vi "PH_IEEE1394Camera.get Cam Video Modes.vi"(0 "i ref in":refnum<vi>, 2 "IMAQ1394 Session In":T1, 4 "Cam Error in":errorcluster, 5 "error in (no error)":errorcluster) -> (14 "i ref out":refnum<vi>, 16 "IMAQ1394 Session Out":T1, 18 "Cam Error out":errorcluster, 19 "error out":errorcluster)   [LabVIEW 2014, in "PH_IEEE1394Camera.lvlib"]
doc: "This VI gets the video modes and sets them to the GUI and own attributes."
uses:
  PH_IEEE1394Camera.lvlib
  <vilib>/userdefined/High Color/IMAQdx.ctl
  <vilib>/vision/driver/NI_Vision_Acquisition_Software.lvlib
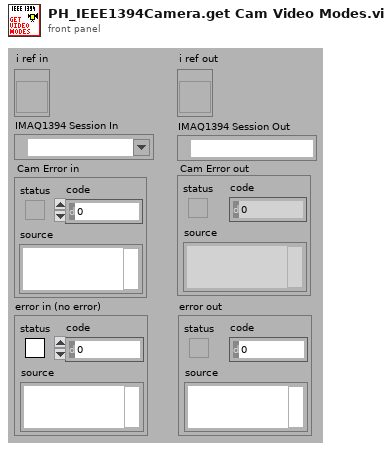
[diagram p1: front panel]
types:
  T1 = typedef "IMAQdx.ctl" = refnum<k21>
  T2 = cluster{"Video Mode":u32, "Video Mode Name":string}[]
  T3 = typedef "PH_IEEE1394Camera.lvlib/PH_IEEE1394Camera.i attribute.ctl" = cluster{"Gui Refs":cluster{"Brightness":refnum<vi>, "Shutter":refnum<vi>, "Gain":refnum<vi>, "Center of Gravity":refnum<vi>, "Supported Video Modes":refnum<vi>, "Trigger Polarity":refnum<vi>, "Trigger Mode":refnum<vi>, "Trigger Timeout":refnum<vi>, "Bit Depth":refnum<vi>, "Video Mode":refnum<vi>, "Top":refnum<vi>, "Bottom":refnum<vi>, "Left":refnum<vi>, "Right":refnum<vi>, "Set ROI to Maximum":refnum<vi>, "Camera Details":refnum<vi>, "Current Cam Attributes":refnum<vi>, "Attribute to set":refnum<vi>, "Num Value":refnum<vi>, "String Value":refnum<vi>, "Bool Value":refnum<vi>, "Set Cam Attribute":refnum<vi>}, "Cam":cluster{"IMAQ1394 Session":T1, "Camera Details":T4}, "Current Attributes":T5[], "Supported Video Modes ":cluster{"Video Mode":u32, "Video Mode Name":string}[], "Wanted Attributes":cluster{"Name":string, "Num Value":dbl, "String Value":string, "Boolean Value":bool}[], "Cam Attributes":T7}
  T4 = typedef "PH_IEEE1394Camera.lvlib/PH_IEEE1394Camera.Cam Details.ctl" = cluster{"Model":string, "Serial Number":dbl, "Cam name (Machinery)":string, "Bus Type":string}
  T5 = typedef "PH_IEEE1394Camera.lvlib/PH_IEEE1394Camera.Cam Attribute.ctl" = cluster{"Information":cluster{"Type":T6, "Readable":bool, "Writable":bool, "Name":string}, "Num Value":dbl, "String Value":string, "Maximum":dbl, "Minimum":dbl, "Units":string, "Description":string, "EnumStrings[]":string[], "EnumValues[]":u32[], "Boolean Value":bool}
  T6 = typedef "NI_Vision_Acquisition_Software.lvlib/IMAQdx Attribute Type.ctl" = enum32{"U32", "I64", "DBL", "String", "Enum", "Bool", "Command"}
  T7 = typedef "PH_IEEE1394Camera.lvlib/PH_IEEE1394Camera.Relevant Cam Attributes.ctl" = cluster{"Video Mode":cluster{"Name":string, "Index":i32}, "Brightness":cluster{"Name":string, "Index":i32}, "Gain":cluster{"Name":string, "Index":i32}, "Shutter":cluster{"Name":string, "Index":i32}, "Trigger Pol":cluster{"Name":string, "Index":i32}, "Trigger Mode":cluster{"Name":string, "Index":i32}, "Timeout":cluster{"Name":string, "Index":i32}, "Bit Depth":cluster{"Name":string, "Index":i32}, "Pixel Bits":cluster{"Name":string, "Index":i32}, "Pixel Bytes":cluster{"Name":string, "Index":i32}, "Left":cluster{"Name":string, "Index":i32}, "Right":cluster{"Name":string, "Index":i32}, "Top":cluster{"Name":string, "Index":i32}, "Bottom":cluster{"Name":string, "Index":i32}}
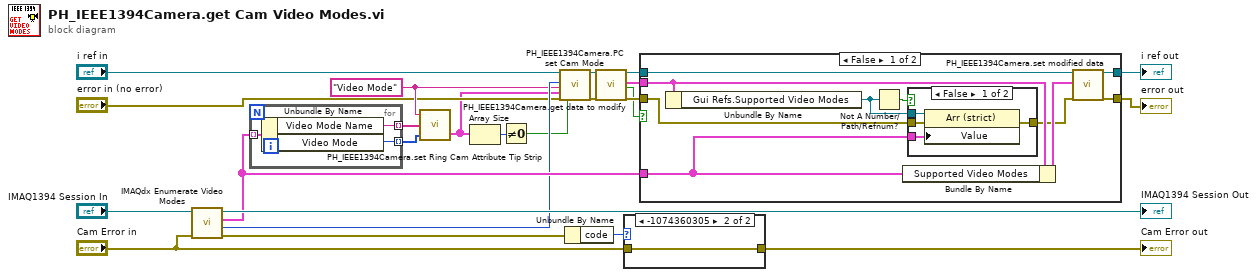
[diagram p0: block diagram]
diagram:
  w9 = "Video Mode" ("Attribute Name")
  n1 = call <vilib>:"IMAQdx Enumerate Video Modes.vi"("error in"="Cam Error in", "Session In"="IMAQ1394 Session In") -> ("error out"=w5:errorcluster, "Current Mode"=w10:u32, "Video Modes"=w11:T2, "Session Out"=→"IMAQ1394 Session Out":T1)  [unwired: 6 in]
  n2 = for {
    tunnel: w11 -> [w27] mode=indexing
    tunnel: [w26] -> w16 mode=indexing
    tunnel: [w25] -> w17 mode=indexing
    n3 = Unbundle By Name(w27) -> ("Video Mode Name"=w26:string, "Video Mode"=w25:u32)
  }
  n4 = call "PH_IEEE1394Camera.set Ring Cam Attribute Tip Strip.vi"("EnumValues[]"=w17, "EnumStrings[]"=w16, "Attribute Name"=w9) -> ("Strings and Values"=w3:cluster{"String":string, "Value":u32}[])  [unwired: 1 out]
  n5 = Array Size(array=w3) -> (size(s)=w2:i32)
  n6 = Not Equal To 0?(x=w2) -> (x != 0?=w1:bool)
  n7 = call "PH_IEEE1394Camera.PC set Cam Mode.vi"("i ref in"="i ref in", "Video Mode"=w10, "Tip Strip [Empty]"=w9, "Strings And Values [Empty]"=w3, "error in (no error)"="error in (no error)", "GUI element visible (true)"=w1) -> ("i ref out"=w13:refnum<vi>, "error out"=w12:errorcluster)  [unwired: 12 in]
  n8 = Unbundle By Name(w5) -> ("code"=w7:i32)
  n9 = call "PH_IEEE1394Camera.get data to modify.vi"("i ref in"=w13, "error in (no error)"=w12) -> ("i ref out"=w23:refnum<vi>, "i attribute"=w20:T3, "timed out"=w19:bool, "error out"=w24:errorcluster)  [unwired: 14 in]
  n10 = case shown="-1074360305" w7 {
    tunnel: "Cam Error in" -> [w28 w29]
    tunnel: [w28 w29] -> w4
    frame Default {
    }
    frame -1074360305 {
    }
  }
  "Cam Error out" <- w4
  n11 = case shown="False" w19 {
    tunnel: w24 -> [w32 w45]
    tunnel: w23 -> [w30 w46]
    tunnel: [w38 w45] -> w22
    tunnel: [w37 w46] -> w21
    tunnel: w20 -> [w36 _]
    tunnel: w11 -> [w31 _]
    frame False {
      n12 = Unbundle By Name(w36) -> ("Gui Refs.Supported Video Modes"=w34:refnum<vi>)
      n13 = Not A Number/Path/Refnum?(number/path/refnum=w34) -> (NaN/Path/Refnum?=w35:bool)
      n14 = Bundle By Name(cluster=w36, "Supported Video Modes"=w31) -> (w39:T3)
      n15 = case shown="False" w35 {
        tunnel: w34 -> [w43 _]
        tunnel: w32 -> [w42 w44]
        tunnel: [w41 w44] -> w33
        tunnel: w31 -> [w40 _]
        frame False {
          n16 = property class="Arr (strict)"(reference=w43, error in=w42, "Value"=w40) -> (error out=w41:errorcluster)  [unwired: 1 out]
        }
        frame True {
        }
      }
      n17 = call "PH_IEEE1394Camera.set modified data.vi"("i ref in"=w30, "i attribute"=w39, "error in (no error)"=w33) -> ("i ref out"=w37:refnum<vi>, "error out"=w38:errorcluster)  [unwired: 15 in]
    }
    frame True {
    }
  }
  "error out" <- w22
  "i ref out" <- w21
